vi "IMAQ FPGA CXP 8-Bit x 8.vi"(6 "Ready for Output":bool=TRUE, 7 "Reset":bool, 9 "Image Skip Count":u16, 10 "CXP Options":T1, 11 "CXP NI AXI4-S Bus":T3) -> (0 "Output Valid":bool, 2 "Acquisition Status":T2, 3 "Vision Pixel Bus Out":T4={"Pixel Data"=[0, 0, 0, 0, 0, 0, 0, 0], "DV"=[FALSE, FALSE, FALSE, FALSE, FALSE, FALSE, FALSE, FALSE], "EOL"=FALSE, "EOI"=FALSE, "Data Type"=enum."U8 x 8"}, 4 "Ready For Input":bool)   [LabVIEW 2020]
doc: "Acquires images from a CoaXPress camera. The VI converts the pixels from NI_AXI4-S format to a Vision Pixel Bus containing 8 adjacent pixels. The <B>Vision Pixel Bus Out</B> can be connected to Vision FPGA algorithms for processing or transferred to the host. Ensure that this VI is called from a Single Cycle Timed Loop. Use multiple instances of this VI along with <B>Device ID</B> and <B>Stream ID</B> inputs to output a Vision Pixel Bus for multiple cameras."
uses:
  <vilib>/visionFPGA/Controls/IMAQ FPGA Pixel Bus u8x8.ctl
  <vilib>/visionFPGA/Basics/CoaXPress Acquisition/Controls/IMAQ FPGA CXP NI AXI4-S Bus.ctl
  <vilib>/visionFPGA/Basics/CoaXPress Acquisition/Controls/IMAQ FPGA CXP FPGA Options.ctl
  <vilib>/rvi/Emulation/niFpgaSctlEmulationGetInTimedLoop.vi
  <vilib>/Utility/error.llb/Clear Errors.vi
  <vilib>/rvi/DataTransferAndStorage/Container/Common/niFpgaContainerGetUniqueNameForEmu.vi
  <vilib>/rvi/DataTransferAndStorage/Container/Common/niFpgaContainerSetEmuInfo.vi
  <vilib>/rvi/eio/common/nirviEmuReportErrorAndStop.vi
  <vilib>/rvi/DataTransferAndStorage/Container/Common/niFpgaContainerExecOnDevCompGetState.vi
  <vilib>/rvi/Emulation/niFpgaEmulationIsFPGAContextNoSignature.vi
  <vilib>/rvi/errors/niFpgaSetErrorForExecOnDevCompSimple.vi
  <vilib>/rvi/FIFO/Fifo_Resource/nirvififoEmulationSetSize.vi
  <vilib>/rvi/FIFO/Fifo_Resource/nirviFifoEmulationQueueMgr.vi
  <instcachedir>/0/nirviFifoEmulationQueueMgr_E5CAEC123FF24DC58D834DCA3CDAA9B5.lvgen/nirviFifoEmulationQueueMgr_E5CAEC123FF24DC58D834DCA3CDAA9B5_008.vi
  <vilib>/rvi/FIFO/Fifo_Resource/nirvififoEmulationDetermineInputValidOut.vi
  <vilib>/rvi/FIFO/Fifo_Resource/nirvififoEmulationCreateLock.vi
  <vilib>/rvi/Emulation/niFpgaProcessEmulError.vi
  <vilib>/rvi/FIFO/Fifo_Resource/nirvififoEmulationObtainLock.vi
  <vilib>/rvi/FIFO/Fifo_Resource/nirvififoEmulationReleaseLock.vi
  <vilib>/rvi/occurrence/nirviWaitOnOccurrenceBase.vi
  <vilib>/rvi/errors/nirviReportUnexpectedCaseInternalError.vi
  <vilib>/rvi/errors/nirviReportUnexpectedCaseInternalError (U32).vi
  <vilib>/rvi/interface/RandomDataEmulation/niFpgaRandomDataHandleErrors.vi
  <vilib>/rvi/LocalResourceManager/LocalResourceManager.xnode
  <vilib>/rvi/DataTransferAndStorage/Container/XNode/niFpgaContainer.xnode
  <vilib>/rvi/FIFO/Fifo_Resource/niFpgaFifoEmulationRefIn.vi
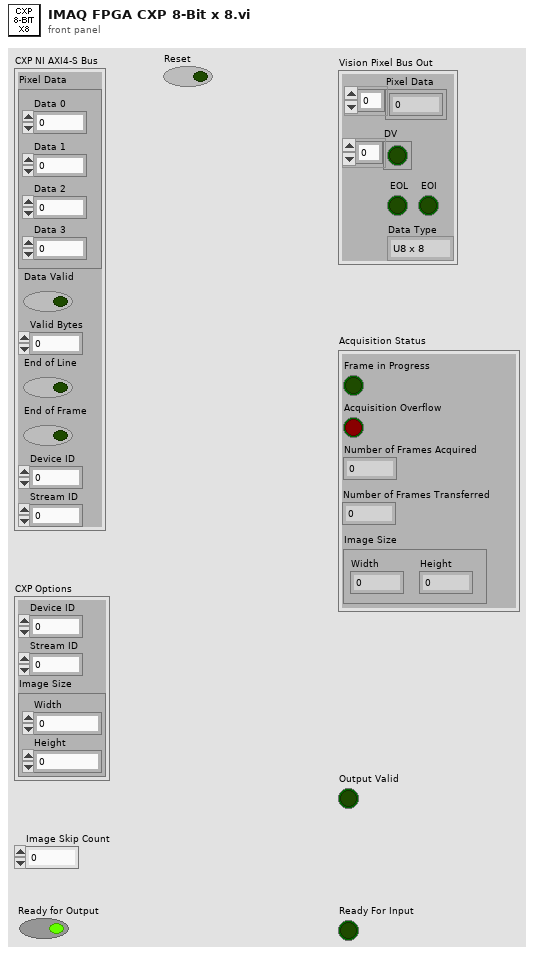
[diagram p1: front panel]
types:
  T1 = typedef "IMAQ FPGA CXP FPGA Options.ctl" = cluster{"Device ID":u8, "Stream ID":u8, "Image Size":cluster{"Width":u16, "Height":u16}}
  T2 = cluster{"Frame in Progress":bool, "Acquisition Overflow":bool, "Number of Frames Acquired":u64, "Number of Frames Transferred":u64, "Image Size":cluster{"Width":u16, "Height":u16}}
  T3 = typedef "IMAQ FPGA CXP NI AXI4-S Bus.ctl" = cluster{"Pixel Data":cluster{"Data 0":u64, "Data 1":u64, "Data 2":u64, "Data 3":u64}, "Data Valid":bool, "Valid Bytes":u8, "End of Line":bool, "End of Frame":bool, "Device ID":u8, "Stream ID":u8}
  T4 = typedef "IMAQ FPGA Pixel Bus u8x8.ctl" = cluster{"Pixel Data":u8[], "DV":bool[], "EOL":bool, "EOI":bool, "Data Type":enum16{"U8 x 8"}}
  T5 = cluster{"Pixel Data":cluster{"Data 0":u64, "Data 1":u64, "Data 2":u64, "Data 3":u64}, "Data Valid":bool, "Valid Bytes":u8, "End of Line":bool, "End of Frame":bool, "Device ID":u8, "Stream ID":u8}
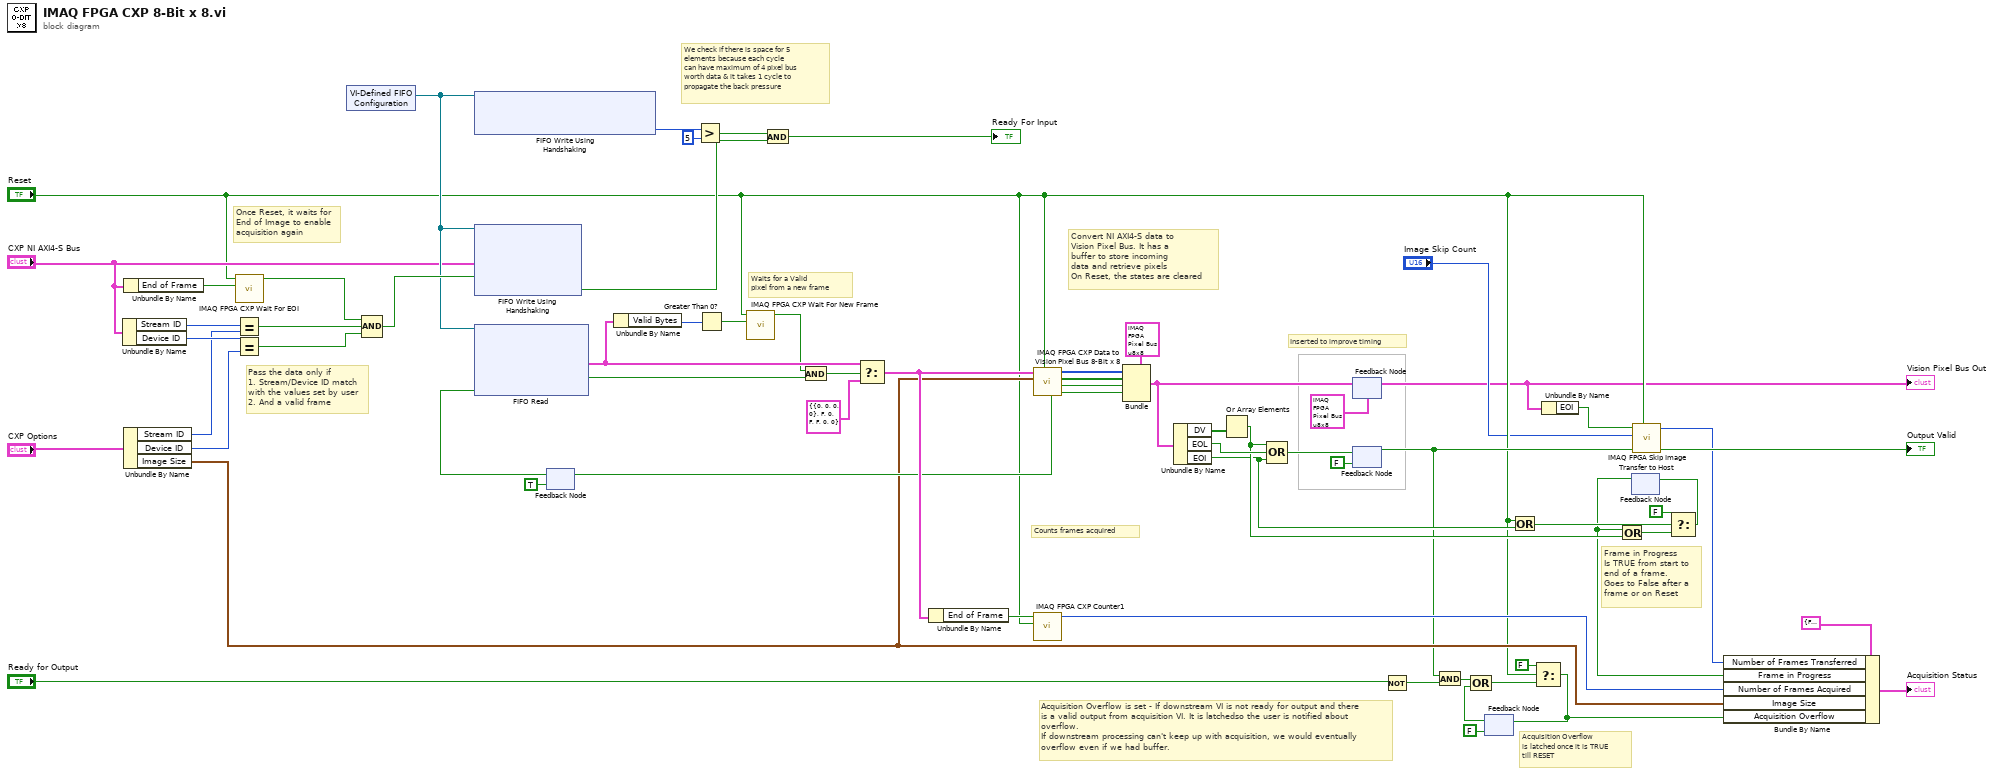
[diagram p0: block diagram]
diagram:
  # "We check if there is space for 5\nelements because each cycle\ncan have maximum of 4 pixel bus\nworth data & it takes 1 cycle to \npropagate the back pressure"
  # "Waits for a Valid\npixel from a new frame"
  # "Once Reset, it waits for\nEnd of Image to enable\nacquisition again"
  # "Frame in Progress\nIs TRUE from start to \nend of a frame. \nGoes to False after a\nframe or on Reset"
  # "Acquisition Overflow\nis latched once it is TRUE\ntill RESET"
  # "Convert NI AXI4-S data to\nVision Pixel Bus. It has a \nbuffer to store incoming\ndata and retrieve pixels\nOn Reset, the states are cleared"
  # "Pass the data only if\n1. Stream/Device ID match\nwith the values set by user\n2. And a valid frame"
  # "Counts frames acquired"
  # "Inserted to improve timing"
  # "Acquisition Overflow is set - If downstream VI is not ready for output and there \nis a valid output from acquisition VI. It is latchedso the user is notified about\noverflow. \nIf downstream processing can't keep up with acquisition, we would eventually \noverflow even if we had buffer."
  n1 = Unbundle By Name("CXP NI AXI4-S Bus") -> ("Stream ID"=w44:u8, "Device ID"=w43:u8)
  n2 = Unbundle By Name("CXP Options") -> ("Stream ID"=w11:u8, "Device ID"=w10:u8, "Image Size"=w12:cluster{"Width":u16, "Height":u16})
  n3 = Unbundle By Name("CXP NI AXI4-S Bus") -> ("End of Frame"=w25:bool)
  n4 = call <vilib>:"IMAQ FPGA CXP Wait For EOI.vi"("EOI"=w25, "Reset"="Reset") -> ("Enable"=w23:bool)  [unwired: 9 in]
  n5 = Equal?(x=w44, y=w11) -> (x = y?=w51:bool)
  n6 = Equal?(x=w43, y=w10) -> (x = y?=w50:bool)
  n7 = xnode "VI-Defined FIFO Configuration"() -> ("FIFO Out"=w35:refnum<k21>)
  n8 = Compound Arithmetic op=AND(w23, w51, w50) -> (w39:bool)
  n9 = xnode "FIFO Write Using Handshaking"("FIFO In"=w35) -> ("Number of Elements to Write"=w34:u32)  [unwired: 1 out]
  n10 = xnode "FIFO Write Using Handshaking"("Element"="CXP NI AXI4-S Bus", "Input Valid"=w39, "FIFO In"=w35) -> ("Ready for Input"=w15:bool)  [unwired: 1 out]
  n11 = feedback #1(TRUE ("Ready for Input")) -> (w38:bool)
  n12 = xnode "FIFO Read"("Ready for Output"=w38, "FIFO In"=w35) -> ("Element"=w22:T5, "Output Valid"=w18:bool)  [unwired: 1 out]
  n13 = Unbundle By Name(w22) -> ("Valid Bytes"=w21:u8)
  n14 = Greater?(x=w34, y=u32 5) -> (0:w16:bool)
  n15 = Greater Than 0?(x=w21) -> (x > 0?=w20:bool)
  n16 = call <vilib>:"IMAQ FPGA CXP Wait For New Frame.vi"("DV"=w20, "Reset"="Reset") -> ("Enable"=w19:bool)  [unwired: 9 in]
  n17 = And(x=w16, y=w15) -> (x .and. y?=→"Ready For Input":bool)
  n18 = And(x=w19, y=w18) -> (x .and. y?=w17:bool)
  n19 = Select(t=w22, s=w17, f=T3 {"Pixel Data"={"Data 0"=0, "Data 1"=0, "Data 2"=0, "Data 3"=0}, "Data Valid"=FALSE, "Valid Bytes"=0, "End of Line"=FALSE, "End of Frame"=FALSE, "Device ID"=0, "Stream ID"=0} ("CXP NI AXI4-S Bus")) -> (s? t:f=w45:T3)
  n20 = Unbundle By Name(w45) -> ("End of Frame"=w47:bool)
  n21 = call <vilib>:"IMAQ FPGA CXP Data to Vision Pixel Bus 8-Bit x 8.vi"("Reset"="Reset", "Image Size"=w12, "CXP Data"=w45) -> ("EOI"=w60:bool, "EOL"=w61:bool, "DV"=w62:bool[], "Pixel Data"=w63:u8[], "Ready for Input"=w37:bool)  [unwired: 4 in]
  n22 = feedback-in #1(w37) -> ()
  n23 = call <vilib>:"IMAQ FPGA CXP Counter1.vi"("Reset"="Reset", "Increment"=w47) -> ("Count 1"=w46:u64)  [unwired: 9 in]
  n24 = Bundle(cluster=T4 {"Pixel Data"=[0, 0, 0, 0, 0, 0, 0, 0], "DV"=[FALSE, FALSE, FALSE, FALSE, FALSE, FALSE, FALSE, FALSE], "EOL"=FALSE, "EOI"=FALSE, "Data Type"=enum."U8 x 8"} ("Pixel Bus In 2"), "Pixel Data"=w63, "DV"=w62, "EOL"=w61, "EOI"=w60) -> (w59:T4)  [unwired: 1 in]
  n25 = Unbundle By Name(w59) -> ("DV"=w65:bool[], "EOL"=w66:bool, "EOI"=w28:bool)
  n26 = Or Array Elements(Boolean array=w65) -> (logical OR=w29:bool)
  n27 = Compound Arithmetic op=OR(w29, w66, w28) -> (w58:bool)
  n28 = feedback #2(T4 {"Pixel Data"=[0, 0, 0, 0, 0, 0, 0, 0], "DV"=[FALSE, FALSE, FALSE, FALSE, FALSE, FALSE, FALSE, FALSE], "EOL"=FALSE, "EOI"=FALSE, "Data Type"=enum."U8 x 8"} ("Pixel Bus In 2")) -> (w5:T4)
  "Vision Pixel Bus Out" <- w5
  n29 = feedback-in #2(w59) -> ()
  n30 = feedback #3(FALSE) -> (w9:bool)
  n31 = feedback-in #3(w58) -> ()
  n32 = Not(x="Ready for Output") -> (.not. x?=w57:bool)
  n33 = And(x=w9, y=w57) -> (x .and. y?=w56:bool)
  n34 = feedback #4(FALSE ("Reset Overflow")) -> (w48:bool)
  n35 = Compound Arithmetic op=OR(w56, w48) -> (w42:bool)
  n36 = Or(x="Reset", y=w28) -> (x .or. y?=w32:bool)
  n37 = Select(t=FALSE, s="Reset", f=w42) -> (s? t:f=w41:bool)
  n38 = feedback-in #4(w41) -> ()
  n39 = Unbundle By Name(w5) -> ("EOI"=w4:bool)
  n40 = feedback #5() -> (w26:bool)  [unwired: 1 in]
  n41 = Or(x=w26, y=w29) -> (x .or. y?=w30:bool)
  n42 = call <vilib>:"IMAQ FPGA Skip Image Transfer to Host.vi"("Reset"="Reset", "Output Valid In"=w9, "Image Skip Count"="Image Skip Count", "EOI In"=w4) -> ("Output Valid Out"=→"Output Valid":bool, "Number of Frames Transferred"=w3:u64)  [unwired: 6 in]
  n43 = Select(t=FALSE ("x .or. y?"), s=w32, f=w30) -> (s? t:f=w27:bool)
  n44 = feedback-in #5(w27) -> ()
  n45 = Bundle By Name(cluster=T2 {"Frame in Progress"=FALSE, "Acquisition Overflow"=FALSE, "Number of Frames Acquired"=0, "Number of Frames Transferred"=0, "Image Size"={"Width"=0, "Height"=0}} ("Acquisition Status"), "Number of Frames Transferred"=w3, "Frame in Progress"=w26, "Number of Frames Acquired"=w46, "Image Size"=w12, "Acquisition Overflow"=w41) -> (→"Acquisition Status":T2)
